vi "F Dwf Analog Impedance Comp Get.vi"(0 "hdwf":i32, 1 "pohmShortReactance":dbl, 5 "pohmOpenResistance":dbl, 7 "pohmOpenReactance":dbl, 9 "pohmShortResistance":dbl, 11 "error in (no error)":errorcluster) -> (3 "pohmShortReactance out":dbl, 4 "function return":i32, 6 "pohmOpenResistance out":dbl, 8 "pohmOpenReactance out":dbl, 10 "pohmShortResistance out":dbl, 15 "error out":errorcluster)   [LabVIEW 2021, in "Olasdwf.lvlib"]
doc: "DWFAPI int FDwfAnalogImpedanceCompGet(HDWF hdwf, double *pohmOpenResistance, double *pohmOpenReactance, double *pohmShortResistance, double *pohmShortReactance);"
uses:
  Olasdwf.lvlib
  Windows/System32/dwf.dll
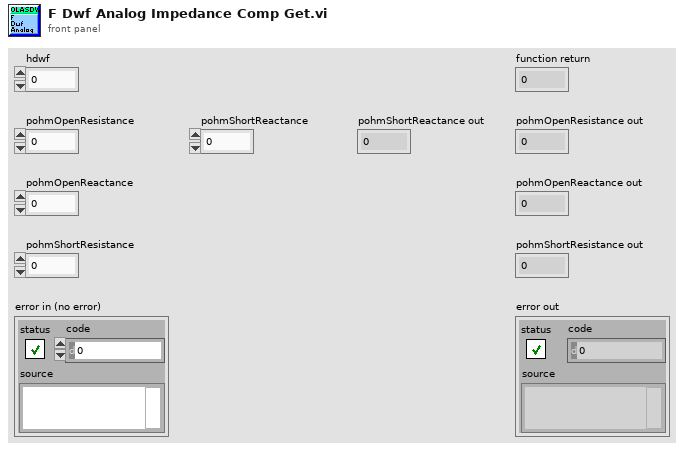
[diagram p1: front panel]
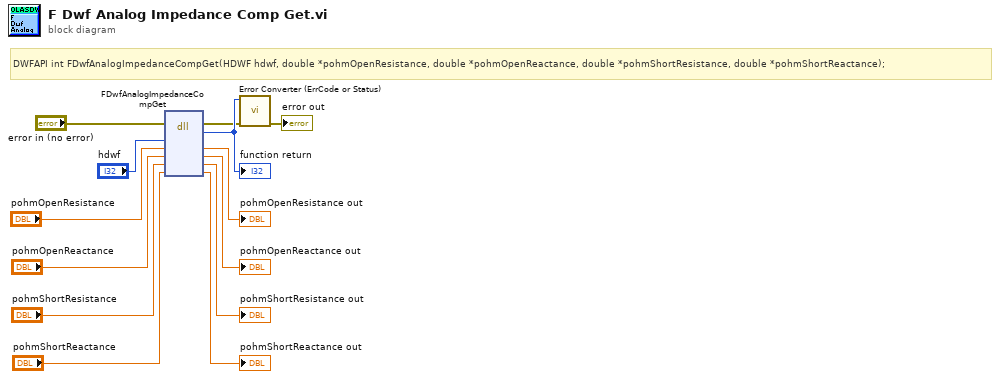
[diagram p0: block diagram]
diagram:
  # "DWFAPI int FDwfAnalogImpedanceCompGet(HDWF hdwf, double *pohmOpenResistance, double *pohmOpenReactance, double *pohmShortResistance, double *pohmShortReactance);"
  n1 = dll-call lib="/Windows/System32/dwf.*" fn="FDwfAnalogImpedanceCompGet"(error in="error in (no error)", "hdwf"="hdwf", "pohmOpenResistance"="pohmOpenResistance", "pohmOpenReactance"="pohmOpenReactance", "pohmShortResistance"="pohmShortResistance", "pohmShortReactance"="pohmShortReactance") -> (error out=w2:errorcluster, w13:i32, "pohmOpenResistance"=→"pohmOpenResistance out":dbl, "pohmOpenReactance"=→"pohmOpenReactance out":dbl, "pohmShortResistance"=→"pohmShortResistance out":dbl, "pohmShortReactance"=→"pohmShortReactance out":dbl)  [unwired: 3 in, 1 out]
  "function return" <- w13
  n2 = call "Error Converter (ErrCode or Status).vi"("error in (no error)"=w2, "error code"=w13) -> ("error out"=→"error out":errorcluster)  [unwired: 9 in]
